vi "Constructor_StartupSplash.vi"(8 "error in (no error)":errorcluster) -> (0 "error out":errorcluster, 3 "StartupSplash out":refnum<class "StartupSplash.lvclass">)   [LabVIEW 2025, in "StartupSplash.lvclass"]
uses:
  StartupSplash.lvclass
  <vilib>/Utility/sysdir.llb/System Directory Type.ctl
  libzmq-v143-mt-4_3_6/ctls/SocketType.ctl
  StartupSplash.lvclass/StartupSplash.ctl
  zeromq/Context.lvclass
  libzmq-v143-mt-4_3_6/LibZMQ.lvlib
  zeromq/Socket.lvclass
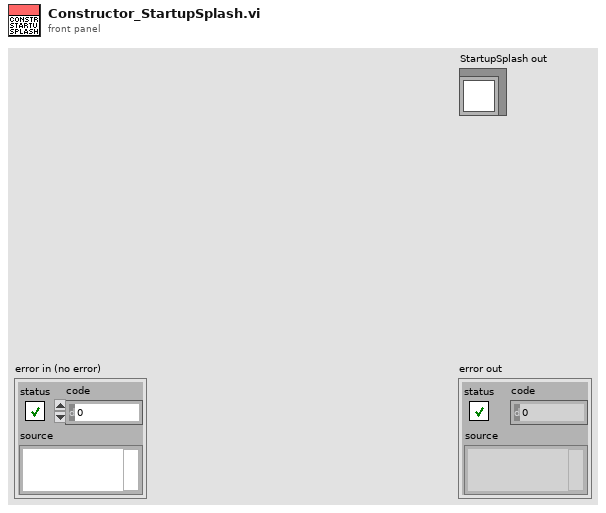
[diagram p1: front panel]
types:
  T1 = typedef "LibZMQ.lvlib/SocketType.ctl" = enum8{"PAIR", "PUB", "SUB", "REQ", "REP", "DEALER", "ROUTER", "PULL", "PUSH", "XPUB", "XSUB", "STREAM"}
  T2 = typedef "System Directory Type.ctl" = i32
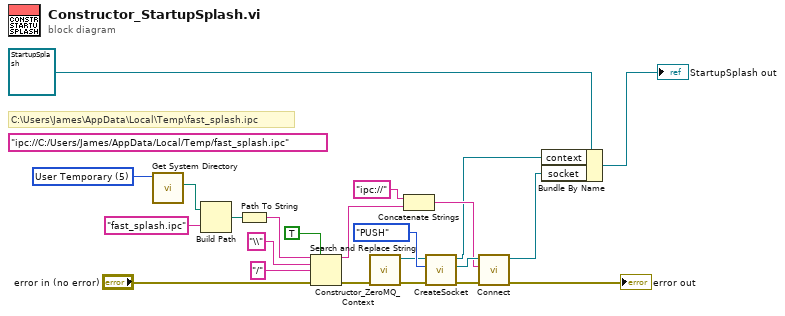
[diagram p0: block diagram]
diagram:
  w23 = T2 5 items=["User Home"=0, "User Desktop"=1, "User Documents"=2, "User Application Data"=3, "User Preferences"=4, "User Temporary"=5, "Public Documents"=6, "Public Application Data"=7, "Public Preferences"=8, "Public Cache"=13, "System Core Libraries"=9, "System Installed Libraries"=10, "Application Files"=11, "Boot Volume Root"=12] ("system directory type")
  (unwired) "ipc://C:/Users/James/AppData/Local/Temp/fast_splash.ipc"
  # "C:\\Users\\James\\AppData\\Local\\Temp\\fast_splash.ipc"
  n1 = call <vilib>:"Get System Directory.vi"("system directory type"=w23) -> ("system directory"=w22:path)  [unwired: 10 in]
  n2 = Build Path(base path=w22, name or relative path="fast_splash.ipc") -> (appended path=w20:path)
  n3 = Path To String(path=w20) -> (string=w19:string)
  n4 = Search and Replace String(replace all?=TRUE ("replace all? (F)"), input string=w19, search string="\\", replace string="/" ("replace string (\"\")"), error in="error in (no error)") -> (result string=w17:string, error out=w8:errorcluster)  [unwired: 3 in, 2 out]
  n5 = call "Constructor_ZeroMQ_Context.vi"("error in"=w8) -> ("error out"=w13:errorcluster, "context out"=w9:refnum<class "Context.lvclass">)  [unwired: 9 in]
  n6 = Concatenate Strings("ipc://" ("string"), w17) -> (w7:string)
  n7 = call "CreateSocket.vi"("error in"=w13, "Socket Type"=SocketType."PUSH", "context in"=w9) -> ("error out"=w11:errorcluster, "socket out"=w12:refnum<class "Socket.lvclass">, "context out"=w4:refnum<class "Context.lvclass">)  [unwired: 6 in]
  n8 = call "Connect.vi"("error in"=w11, "endpoint"=w7, "socket in"=w12) -> ("error out"=→"error out":errorcluster, "socket out"=w3:refnum<class "Socket.lvclass">)  [unwired: 7 in]
  n9 = Bundle By Name(cluster=refnum<class "StartupSplash.lvclass"> refnum ("StartupSplash in"), "context"=w4, "socket"=w3) -> (→"StartupSplash out":refnum<class "StartupSplash.lvclass">)
